vi "loadSignImage.vi"(8 "inputError":errorcluster, 10 "String":string) -> (0 "outputError":errorcluster, 2 "SignImageOutput":picture[](array[picture]))   [LabVIEW 2020]
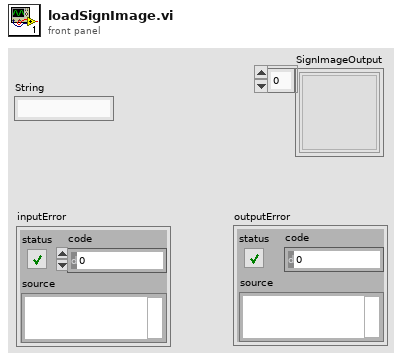
[diagram p1: front panel]
types:
  T1 = typedef "imagedata.ctl" = cluster{"image type":i32, "image depth":i32, "image":u8[], "mask":u8[], "colors":u32[], "Rectangle":cluster{"left":i16, "top":i16, "right":i16, "bottom":i16}}
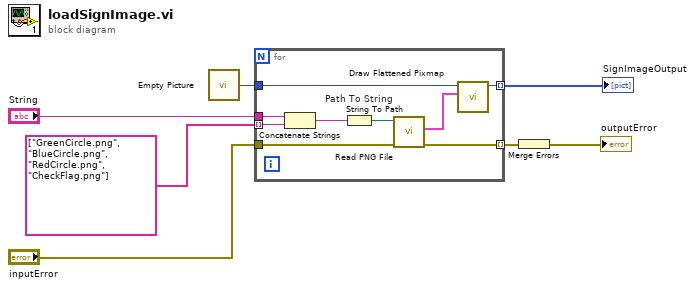
[diagram p0: block diagram]
diagram:
  n1 = call "Empty Picture"() -> ("empty picture"=w4:picture)
  n2 = for {
    tunnel: [w16] -> w6 mode=indexing
    tunnel: [w14] -> w7 mode=indexing
    tunnel: "String" -> [w12]
    tunnel: string[] ["GreenCircle.png", "BlueCircle.png", "RedCircle.png", "CheckFlag.png"] -> [w11] mode=indexing
    tunnel: w4 -> [w9]
    tunnel: "inputError" -> [w8]
    n3 = Concatenate Strings "Concatenate Strings"(w12, w11) -> (w13:string)
    n4 = String To Path "Path To String"(string=w13) -> (path=w10:path)
    n5 = call <vilib>:"Read PNG File.vi"("error in (no error)"=w8, "path to PNG file"=w10) -> ("error out"=w16:errorcluster, "image data"=w15:T1)  [unwired: 7 in, 1 out]
    n6 = call <vilib>:"Draw Flattened Pixmap.vi"("image data"=w15, "picture"=w9) -> ("new picture"=w14:picture)  [unwired: 7 in]
  }
  "SignImageOutput" <- w7
  n7 = Merge Errors "Merge Errors"(w6) -> (→"outputError":errorcluster)
